vi "Read SQLite Library Path.vi"(8 "error in (no error)":errorcluster, 11 "Connection in":refnum<class "Connection.lvclass">) -> (0 "error out":errorcluster, 2 "SQLite Library Path":path, 3 "Connection out":refnum<class "Connection.lvclass">)   [LabVIEW 2023, in "SQLite.lvlib" / "Connection.lvclass"]
doc: "The path to the SQLite3 shared library (DLL on Windows) in use."
uses:
  Connection.lvclass
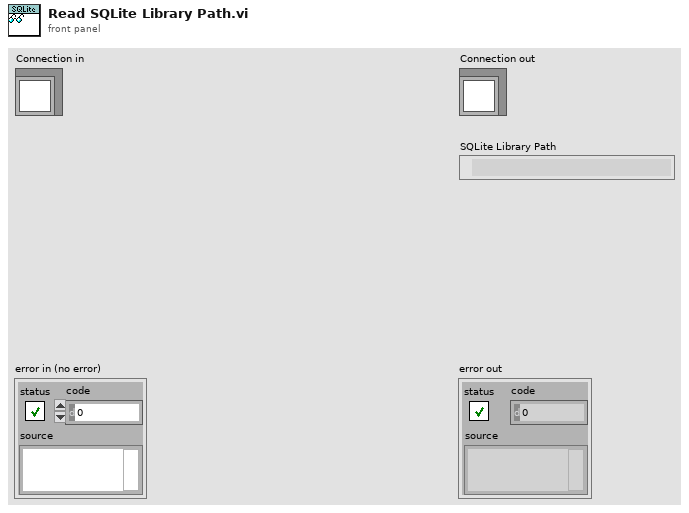
[diagram p1: front panel]
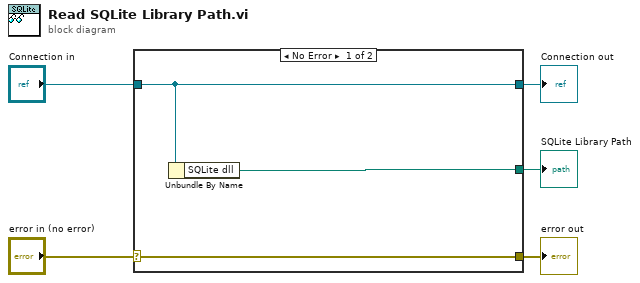
[diagram p0: block diagram]
diagram:
  n1 = case shown="No Error" "error in (no error)" {
    selector: "error in (no error)" -> [w8 w9]
    tunnel: [w8 w9] -> w4
    tunnel: [w7 w10] -> w2
    tunnel: "Connection in" -> [w7 w10]
    tunnel: [w6 _] -> w1
    frame No Error {
      n2 = Unbundle By Name(w7) -> ("SQLite dll"=w6:path)
    }
    frame Error {
    }
  }
  "error out" <- w4
  "Connection out" <- w2
  "SQLite Library Path" <- w1
